vi "LaunchSystemMessageDialogBox.vi"(6 "ErrorToProcess":errorcluster, 7 "SMS":T1, 8 "ErrorIn":errorcluster, 10 "CorrAct":string, 11 "Timeout(ms)":i32=-1) -> (0 "ErrorOut":errorcluster)   [LabVIEW 2018]
uses:
  Controls/SMSDataCluster.ctl
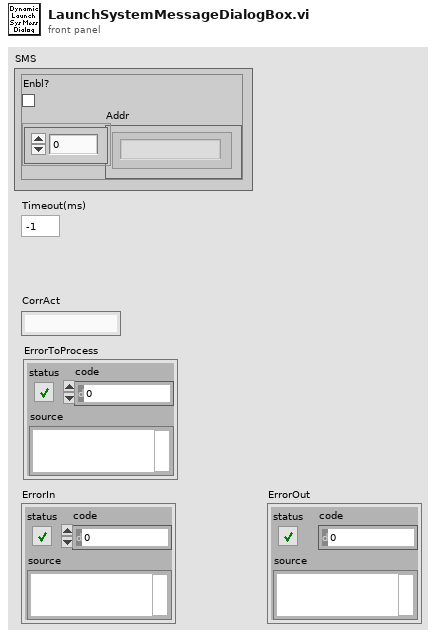
[diagram p1: front panel]
types:
  T1 = typedef "SMSDataCluster.ctl" = cluster{"Enbl?":bool, "Addr":string[]}
  T2 = enum32{"Invalid", "Standard", "Closed", "Hidden", "Minimized", "Maximized"}
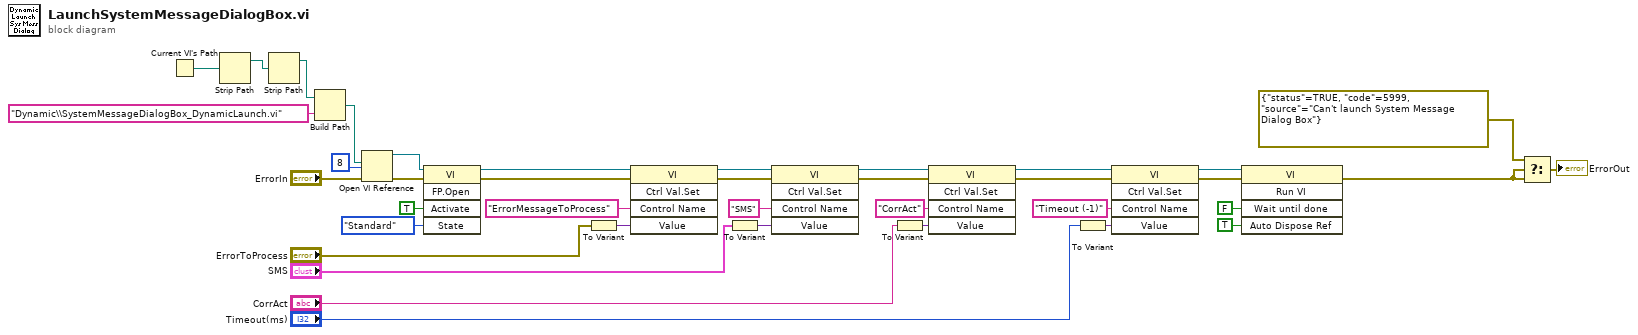
[diagram p0: block diagram]
diagram:
  n1 = Current VI's Path() -> (path=w2:path)
  n2 = Strip Path(path=w2) -> (stripped path=w1:path)  [unwired: 1 out]
  n3 = Strip Path(path=w1) -> (stripped path=w3:path)  [unwired: 1 out]
  n4 = Build Path(base path=w3, name or relative path="Dynamic\\SystemMessageDialogBox_DynamicLaunch.vi") -> (appended path=w28:path)
  n5 = Open VI Reference(vi path=w28, options=8, error in (no error)="ErrorIn") -> (vi reference=w38:refnum<vi>, error out=w37:errorcluster)  [unwired: 3 in]
  n6 = invoke class="VI" method="FP.Open"(reference=w38, error in=w37, "Activate"=TRUE ("Activate?"), "State"=T2."Standard") -> (reference out=w18:refnum<vi>, error out=w19:errorcluster)  [unwired: 1 in, 3 out]
  n7 = To Variant(anything="ErrorToProcess") -> (Variant=w33:variant)
  n8 = invoke class="VI" method="Ctrl Val.Set"(reference=w18, error in=w19, "Control Name"="ErrorMessageToProcess", "Value"=w33) -> (reference out=w11:refnum<vi>, error out=w10:errorcluster)  [unwired: 1 in, 3 out]
  n9 = To Variant(anything="SMS") -> (Variant=w13:variant)
  n10 = invoke class="VI" method="Ctrl Val.Set"(reference=w11, error in=w10, "Control Name"="SMS", "Value"=w13) -> (reference out=w5:refnum<vi>, error out=w4:errorcluster)  [unwired: 1 in, 3 out]
  n11 = To Variant(anything="CorrAct") -> (Variant=w23:variant)
  n12 = invoke class="VI" method="Ctrl Val.Set"(reference=w5, error in=w4, "Control Name"="CorrAct", "Value"=w23) -> (reference out=w22:refnum<vi>, error out=w21:errorcluster)  [unwired: 1 in, 3 out]
  n13 = To Variant(anything="Timeout(ms)") -> (Variant=w27:variant)
  n14 = invoke class="VI" method="Ctrl Val.Set"(reference=w22, error in=w21, "Control Name"="Timeout (-1)", "Value"=w27) -> (reference out=w17:refnum<vi>, error out=w16:errorcluster)  [unwired: 1 in, 3 out]
  n15 = invoke class="VI" method="Run VI"(reference=w17, error in=w16, "Wait until done"=FALSE ("Wait Until Done"), "Auto Dispose Ref"=TRUE ("Auto Dispose Reference")) -> (error out=w7:errorcluster)  [unwired: 1 in, 4 out]
  n16 = Select(t=errorcluster {"status"=TRUE, "code"=5999, "source"="Can't launch System Message Dialog Box"}, s=w7, f=w7) -> (s? t:f=→"ErrorOut":errorcluster)
